vi "PV ActiveLine - ErrorRelayAllocation.vi"(7 "W/R":bool, 8 "Fehler (Eingang)":errorcluster, 9 "Error Relay Allocation":u16(ring) items=["Switches for all errors (default)", "Only unit errors", "Error sensor 1 and unit error", "Error sensor 2 and unit error (TPG 362 only)"], 11 "Referenz in":refnum<visa-resource-name>) -> (0 "Cluster (Ausgang)":errorcluster, 1 "Error Relay Allocation out":u16(ring) items=["Switches for all errors (default)", "Only unit errors", "Error sensor 1 and unit error", "Error sensor 2 and unit error (TPG 362 only)"], 3 "Referenz out":refnum<visa-resource-name>)   [LabVIEW 2013, in "PV ActiveLine.lvlib"]
doc: "ERA - Error Relay Allocation\n\nTransmit: ERA [,a]\nReceive: a\n\nSwitching behaviour error relay,\na =\n0 –> Switches for all errors (default)\n1 –> Only unit errors\n2 –> Error sensor 1 and unit error\n3 –> Error sensor 2 and unit error (TPG 362 only)"
uses:
  <instrlib>/PV ActiveLine/PV ActiveLine.lvlib
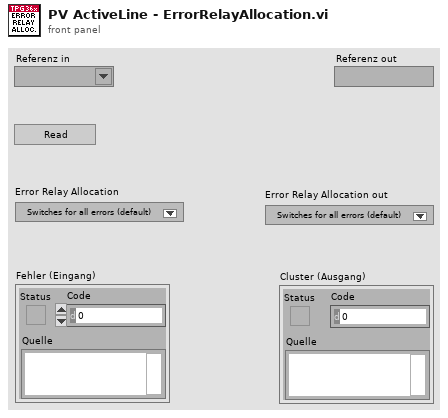
[diagram p1: front panel]
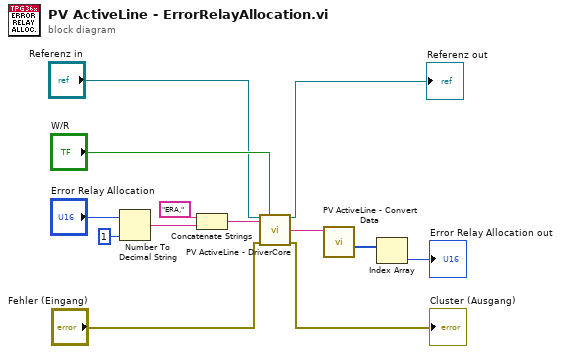
[diagram p0: block diagram]
diagram:
  n1 = Number To Decimal String(number="Error Relay Allocation", width (-)=i16 1 ("Breite (-)")) -> (decimal integer string=w9:string)
  n2 = Concatenate Strings("ERA,", w9) -> (w11:string)
  n3 = call <instrlib>:"PV ActiveLine - DriverCore.vi"("Referenz in"="Referenz in", "Write/Read"="W/R", "Command"=w11, "Fehler (Eingang)"="Fehler (Eingang)") -> ("Referenz out"=→"Referenz out":refnum<visa-resource-name>, "String Out"=w3:string, "Cluster (Ausgang)"=→"Cluster (Ausgang)":errorcluster)  [unwired: 9 in]
  n4 = call <instrlib>:"PV ActiveLine - Convert Data.vi"("String in"=w3) -> ("Integer Out"=w2:i32[])  [unwired: 7 in, 3 out]
  n5 = Index Array(array=w2) -> (element=→"Error Relay Allocation out":i32)  [unwired: 1 in]
